vi "Sort Alarms.vi"(11 "alarms":T2(array[cluster])=[{"alarm URL"="\\\\Nate-VM-LV2018\\Pfizer_FAST_20190308T120351\\TT1.Alarms.TT1:Hi", "set time"=timestamp(3634909448.9887314 s since 1904-01-01), "set user"="(Nobody)", "ack time"=timestamp(-9223372036854775808 s since 1904-01-01), "ack user"="", "clear time"=timestamp(3634909450.4573107 s since 1904-01-01), "clear user"="(Nobody)", "setpoint"=70.0, "value"=70.46992251022208, "priority"=1, "alarm area"="", "alarm description"="", "ack comment"="", "event?"=FALSE, "Refnum"=216172782113784118}, {"alarm URL"="\\\\Nate-VM-LV2018\\Pfizer_FAST_20190308T120351\\TT1.Alarms.TT1:Hi", "set time"=timestamp(3634909451.127358 s since 1904-01-01), "set user"="(Nobody)", "ack time"=timestamp(-9223372036854775808 s since 1904-01-01), "ack user"="", "clear time"=timestamp(3634909453.4071665 s since 1904-01-01), "clear user"="(Nobody)", "setpoint"=70.0, "value"=71.57929385818943, "priority"=1, "alarm area"="", "alarm description"="", "ack comment"="", "event?"=FALSE, "Refnum"=216172782113784119}, {"alarm URL"="\\\\Nate-VM-LV2018\\Pfizer_FAST_20190308T120351\\TT1.Alarms.TT1:Hi", "set time"=timestamp(3634909453.907706 s since 1904-01-01), "set user"="(Nobody)", "ack time"=timestamp(-9223372036854775808 s since 1904-01-01), "ack user"="", "clear time"=timestamp(3634909456.7766027 s since 1904-01-01), "clear user"="(Nobody)", "setpoint"=70.0, "value"=71.76684506124857, "priority"=1, "alarm area"="", "alarm description"="", "ack comment"="", "event?"=FALSE, "Refnum"=216172782113784120}, {"alarm URL"="\\\\Nate-VM-LV2018\\Pfizer_FAST_20190308T120351\\TT1.Alarms.TT1:HiHi", "set time"=timestamp(3634909455.1962986 s since 1904-01-01), "set user"="(Nobody)", "ack time"=timestamp(-9223372036854775808 s since 1904-01-01), "ack user"="", "clear time"=timestamp(3634909456.1466627 s since 1904-01-01), "clear user"="(Nobody)", "setpoint"=80.0, "value"=80.61428399459591, "priority"=100, "alarm area"="", "alarm description"="", "ack comment"="", "event?"=FALSE, "Refnum"=216172782113784121}, {"alarm URL"="\\\\Nate-VM-LV2018\\Pfizer_FAST_20190308T120351\\TT1.Alarms.TT1:Hi", "set time"=timestamp(3634909457.266568 s since 1904-01-01), "set user"="(Nobody)", "ack time"=timestamp(-9223372036854775808 s since 1904-01-01), "ack user"="", "clear time"=timestamp(3634909458.256423 s since 1904-01-01), "clear user"="(Nobody)", "setpoint"=70.0, "value"=74.55000777818069, "priority"=1, "alarm area"="", "alarm description"="", "ack comment"="", "event?"=FALSE, "Refnum"=216172782113784122}, {"alarm URL"="\\\\Nate-VM-LV2018\\Pfizer_FAST_20190308T120351\\TT1.Alarms.TT1:HiHi", "set time"=timestamp(3634909457.306495 s since 1904-01-01), "set user"="(Nobody)", "ack time"=timestamp(-9223372036854775808 s since 1904-01-01), "ack user"="", "clear time"=timestamp(3634909457.716528 s since 1904-01-01), "clear user"="(Nobody)", "setpoint"=80.0, "value"=81.63729425968472, "priority"=100, "alarm area"="", "alarm description"="", "ack comment"="", "event?"=FALSE, "Refnum"=216172782113784123}, {"alarm URL"="\\\\Nate-VM-LV2018\\Pfizer_FAST_20190308T120351\\TT1.Alarms.TT1:HiHi", "set time"=timestamp(3634909457.9566164 s since 1904-01-01), "set user"="(Nobody)", "ack time"=timestamp(-9223372036854775808 s since 1904-01-01), "ack user"="", "clear time"=timestamp(3634909458.186914 s since 1904-01-01), "clear user"="(Nobody)", "setpoint"=80.0, "value"=80.37585970760009, "priority"=100, "alarm area"="", "alarm description"="", "ack comment"="", "event?"=FALSE, "Refnum"=216172782113784124}, {"alarm URL"="\\\\Nate-VM-LV2018\\Pfizer_FAST_20190308T120351\\TT1.Alarms.TT1:Hi", "set time"=timestamp(3634909458.776946 s since 1904-01-01), "set user"="(Nobody)", "ack time"=timestamp(-9223372036854775808 s since 1904-01-01), "ack user"="", "clear time"=timestamp(-9223372036854775808 s since 1904-01-01), "clear user"="", "setpoint"=70.0, "value"=71.54470210070821, "priority"=1, "alarm area"="", "alarm description"="", "ack comment"="", "event?"=FALSE, "Refnum"=216172782113784125}, {"alarm URL"="\\\\Nate-VM-LV2018\\Pfizer_FAST_20190308T120351\\TT1.Alarms.TT1:HiHi", "set time"=timestamp(3634909459.176953 s since 1904-01-01), "set user"="(Nobody)", "ack time"=timestamp(-9223372036854775808 s since 1904-01-01), "ack user"="", "clear time"=timestamp(3634909459.3466263 s since 1904-01-01), "clear user"="(Nobody)", "setpoint"=80.0, "value"=81.23368917949773, "priority"=100, "alarm area"="", "alarm description"="", "ack comment"="", "event?"=FALSE, "Refnum"=216172782113784126}, {"alarm URL"="\\\\Nate-VM-LV2018\\Pfizer_FAST_20190308T120351\\TT2.Alarms.TT2:Lo", "set time"=timestamp(3634909460.636917 s since 1904-01-01), "set user"="(Nobody)", "ack time"=timestamp(-9223372036854775808 s since 1904-01-01), "ack user"="", "clear time"=timestamp(3634909465.4269753 s since 1904-01-01), "clear user"="(Nobody)", "setpoint"=50.0, "value"=47.30826157706679, "priority"=1, "alarm area"="", "alarm description"="", "ack comment"="", "event?"=FALSE, "Refnum"=216172782113784127}, {"alarm URL"="\\\\Nate-VM-LV2018\\Pfizer_FAST_20190308T120351\\TT2.Alarms.TT2:LoLo", "set time"=timestamp(3634909461.5767922 s since 1904-01-01), "set user"="(Nobody)", "ack time"=timestamp(-9223372036854775808 s since 1904-01-01), "ack user"="", "clear time"=timestamp(3634909462.0770683 s since 1904-01-01), "clear user"="(Nobody)", "setpoint"=10.0, "value"=8.506791891117093, "priority"=100, "alarm area"="", "alarm description"="", "ack comment"="", "event?"=FALSE, "Refnum"=216172782113784128}, {"alarm URL"="\\\\Nate-VM-LV2018\\Pfizer_FAST_20190308T120351\\TT2.Alarms.TT2:LoLo", "set time"=timestamp(3634909462.2569776 s since 1904-01-01), "set user"="(Nobody)", "ack time"=timestamp(-9223372036854775808 s since 1904-01-01), "ack user"="", "clear time"=timestamp(3634909462.497084 s since 1904-01-01), "clear user"="(Nobody)", "setpoint"=10.0, "value"=4.924754519008068, "priority"=100, "alarm area"="", "alarm description"="", "ack comment"="", "event?"=FALSE, "Refnum"=216172782113784129}, {"alarm URL"="\\\\Nate-VM-LV2018\\Pfizer_FAST_20190308T120351\\TT2.Alarms.TT2:LoLo", "set time"=timestamp(3634909464.4868274 s since 1904-01-01), "set user"="(Nobody)", "ack time"=timestamp(-9223372036854775808 s since 1904-01-01), "ack user"="", "clear time"=timestamp(3634909464.6469216 s since 1904-01-01), "clear user"="(Nobody)", "setpoint"=10.0, "value"=8.582095188618679, "priority"=100, "alarm area"="", "alarm description"="", "ack comment"="", "event?"=FALSE, "Refnum"=216172782113784130}, {"alarm URL"="\\\\Nate-VM-LV2018\\Pfizer_FAST_20190308T120351\\TT2.Alarms.TT2:LoLo", "set time"=timestamp(3634909464.886837 s since 1904-01-01), "set user"="(Nobody)", "ack time"=timestamp(-9223372036854775808 s since 1904-01-01), "ack user"="", "clear time"=timestamp(3634909465.0468464 s since 1904-01-01), "clear user"="(Nobody)", "setpoint"=10.0, "value"=5.034174395850155, "priority"=100, "alarm area"="", "alarm description"="", "ack comment"="", "event?"=FALSE, "Refnum"=216172782113784131}] {"value" format="%.2f"; "setpoint" format="%.2f"; "clear time" format="%<%X\n%x>T"; "ack time" format="%<%X\n%x>T"; "set time" format="%<%X\n%x>T"}) -> (3 "alarms out":T2(array[cluster])=[{"alarm URL"="\\\\Nate-VM-LV2018\\Pfizer_FAST_20190308T120351\\TT1.Alarms.TT1:Hi", "set time"=timestamp(3634909458.776946 s since 1904-01-01), "set user"="(Nobody)", "ack time"=timestamp(-9223372036854775808 s since 1904-01-01), "ack user"="", "clear time"=timestamp(-9223372036854775808 s since 1904-01-01), "clear user"="", "setpoint"=70.0, "value"=71.54470210070821, "priority"=1, "alarm area"="", "alarm description"="", "ack comment"="", "event?"=FALSE, "Refnum"=216172782113784125}, {"alarm URL"="\\\\Nate-VM-LV2018\\Pfizer_FAST_20190308T120351\\TT2.Alarms.TT2:LoLo", "set time"=timestamp(3634909464.886837 s since 1904-01-01), "set user"="(Nobody)", "ack time"=timestamp(-9223372036854775808 s since 1904-01-01), "ack user"="", "clear time"=timestamp(3634909465.0468464 s since 1904-01-01), "clear user"="(Nobody)", "setpoint"=10.0, "value"=5.034174395850155, "priority"=100, "alarm area"="", "alarm description"="", "ack comment"="", "event?"=FALSE, "Refnum"=216172782113784131}, {"alarm URL"="\\\\Nate-VM-LV2018\\Pfizer_FAST_20190308T120351\\TT2.Alarms.TT2:LoLo", "set time"=timestamp(3634909464.4868274 s since 1904-01-01), "set user"="(Nobody)", "ack time"=timestamp(-9223372036854775808 s since 1904-01-01), "ack user"="", "clear time"=timestamp(3634909464.6469216 s since 1904-01-01), "clear user"="(Nobody)", "setpoint"=10.0, "value"=8.582095188618679, "priority"=100, "alarm area"="", "alarm description"="", "ack comment"="", "event?"=FALSE, "Refnum"=216172782113784130}, {"alarm URL"="\\\\Nate-VM-LV2018\\Pfizer_FAST_20190308T120351\\TT2.Alarms.TT2:LoLo", "set time"=timestamp(3634909462.2569776 s since 1904-01-01), "set user"="(Nobody)", "ack time"=timestamp(-9223372036854775808 s since 1904-01-01), "ack user"="", "clear time"=timestamp(3634909462.497084 s since 1904-01-01), "clear user"="(Nobody)", "setpoint"=10.0, "value"=4.924754519008068, "priority"=100, "alarm area"="", "alarm description"="", "ack comment"="", "event?"=FALSE, "Refnum"=216172782113784129}, {"alarm URL"="\\\\Nate-VM-LV2018\\Pfizer_FAST_20190308T120351\\TT2.Alarms.TT2:LoLo", "set time"=timestamp(3634909461.5767922 s since 1904-01-01), "set user"="(Nobody)", "ack time"=timestamp(-9223372036854775808 s since 1904-01-01), "ack user"="", "clear time"=timestamp(3634909462.0770683 s since 1904-01-01), "clear user"="(Nobody)", "setpoint"=10.0, "value"=8.506791891117093, "priority"=100, "alarm area"="", "alarm description"="", "ack comment"="", "event?"=FALSE, "Refnum"=216172782113784128}, {"alarm URL"="\\\\Nate-VM-LV2018\\Pfizer_FAST_20190308T120351\\TT1.Alarms.TT1:HiHi", "set time"=timestamp(3634909459.176953 s since 1904-01-01), "set user"="(Nobody)", "ack time"=timestamp(-9223372036854775808 s since 1904-01-01), "ack user"="", "clear time"=timestamp(3634909459.3466263 s since 1904-01-01), "clear user"="(Nobody)", "setpoint"=80.0, "value"=81.23368917949773, "priority"=100, "alarm area"="", "alarm description"="", "ack comment"="", "event?"=FALSE, "Refnum"=216172782113784126}, {"alarm URL"="\\\\Nate-VM-LV2018\\Pfizer_FAST_20190308T120351\\TT1.Alarms.TT1:HiHi", "set time"=timestamp(3634909457.9566164 s since 1904-01-01), "set user"="(Nobody)", "ack time"=timestamp(-9223372036854775808 s since 1904-01-01), "ack user"="", "clear time"=timestamp(3634909458.186914 s since 1904-01-01), "clear user"="(Nobody)", "setpoint"=80.0, "value"=80.37585970760009, "priority"=100, "alarm area"="", "alarm description"="", "ack comment"="", "event?"=FALSE, "Refnum"=216172782113784124}, {"alarm URL"="\\\\Nate-VM-LV2018\\Pfizer_FAST_20190308T120351\\TT1.Alarms.TT1:HiHi", "set time"=timestamp(3634909457.306495 s since 1904-01-01), "set user"="(Nobody)", "ack time"=timestamp(-9223372036854775808 s since 1904-01-01), "ack user"="", "clear time"=timestamp(3634909457.716528 s since 1904-01-01), "clear user"="(Nobody)", "setpoint"=80.0, "value"=81.63729425968472, "priority"=100, "alarm area"="", "alarm description"="", "ack comment"="", "event?"=FALSE, "Refnum"=216172782113784123}, {"alarm URL"="\\\\Nate-VM-LV2018\\Pfizer_FAST_20190308T120351\\TT1.Alarms.TT1:HiHi", "set time"=timestamp(3634909455.1962986 s since 1904-01-01), "set user"="(Nobody)", "ack time"=timestamp(-9223372036854775808 s since 1904-01-01), "ack user"="", "clear time"=timestamp(3634909456.1466627 s since 1904-01-01), "clear user"="(Nobody)", "setpoint"=80.0, "value"=80.61428399459591, "priority"=100, "alarm area"="", "alarm description"="", "ack comment"="", "event?"=FALSE, "Refnum"=216172782113784121}, {"alarm URL"="\\\\Nate-VM-LV2018\\Pfizer_FAST_20190308T120351\\TT2.Alarms.TT2:Lo", "set time"=timestamp(3634909460.636917 s since 1904-01-01), "set user"="(Nobody)", "ack time"=timestamp(-9223372036854775808 s since 1904-01-01), "ack user"="", "clear time"=timestamp(3634909465.4269753 s since 1904-01-01), "clear user"="(Nobody)", "setpoint"=50.0, "value"=47.30826157706679, "priority"=1, "alarm area"="", "alarm description"="", "ack comment"="", "event?"=FALSE, "Refnum"=216172782113784127}, {"alarm URL"="\\\\Nate-VM-LV2018\\Pfizer_FAST_20190308T120351\\TT1.Alarms.TT1:Hi", "set time"=timestamp(3634909457.266568 s since 1904-01-01), "set user"="(Nobody)", "ack time"=timestamp(-9223372036854775808 s since 1904-01-01), "ack user"="", "clear time"=timestamp(3634909458.256423 s since 1904-01-01), "clear user"="(Nobody)", "setpoint"=70.0, "value"=74.55000777818069, "priority"=1, "alarm area"="", "alarm description"="", "ack comment"="", "event?"=FALSE, "Refnum"=216172782113784122}, {"alarm URL"="\\\\Nate-VM-LV2018\\Pfizer_FAST_20190308T120351\\TT1.Alarms.TT1:Hi", "set time"=timestamp(3634909453.907706 s since 1904-01-01), "set user"="(Nobody)", "ack time"=timestamp(-9223372036854775808 s since 1904-01-01), "ack user"="", "clear time"=timestamp(3634909456.7766027 s since 1904-01-01), "clear user"="(Nobody)", "setpoint"=70.0, "value"=71.76684506124857, "priority"=1, "alarm area"="", "alarm description"="", "ack comment"="", "event?"=FALSE, "Refnum"=216172782113784120}, {"alarm URL"="\\\\Nate-VM-LV2018\\Pfizer_FAST_20190308T120351\\TT1.Alarms.TT1:Hi", "set time"=timestamp(3634909451.127358 s since 1904-01-01), "set user"="(Nobody)", "ack time"=timestamp(-9223372036854775808 s since 1904-01-01), "ack user"="", "clear time"=timestamp(3634909453.4071665 s since 1904-01-01), "clear user"="(Nobody)", "setpoint"=70.0, "value"=71.57929385818943, "priority"=1, "alarm area"="", "alarm description"="", "ack comment"="", "event?"=FALSE, "Refnum"=216172782113784119}, {"alarm URL"="\\\\Nate-VM-LV2018\\Pfizer_FAST_20190308T120351\\TT1.Alarms.TT1:Hi", "set time"=timestamp(3634909448.9887314 s since 1904-01-01), "set user"="(Nobody)", "ack time"=timestamp(-9223372036854775808 s since 1904-01-01), "ack user"="", "clear time"=timestamp(3634909450.4573107 s since 1904-01-01), "clear user"="(Nobody)", "setpoint"=70.0, "value"=70.46992251022208, "priority"=1, "alarm area"="", "alarm description"="", "ack comment"="", "event?"=FALSE, "Refnum"=216172782113784118}] {"value" format="%.2f"; "setpoint" format="%.2f"; "clear time" format="%<%X\n%x>T"; "ack time" format="%<%X\n%x>T"; "set time" format="%<%X\n%x>T"})   [LabVIEW 2018, in "Dynamic Shared Variables.lvlib"]
doc: "Sort alarms per Delta V alarm ranking."
uses:
  Dynamic Shared Variables.lvlib
panel:
  out "Array":T1(array[cluster])=[{113635.90945877694604, "Alarm"={"alarm URL"="\\\\Nate-VM-LV2018\\Pfizer_FAST_20190308T120351\\TT1.Alarms.TT1:Hi", "set time"=timestamp(3634909458.776946 s since 1904-01-01), "set user"="(Nobody)", "ack time"=timestamp(-9223372036854775808 s since 1904-01-01), "ack user"="", "clear time"=timestamp(-9223372036854775808 s since 1904-01-01), "clear user"="", "setpoint"=70.0, "value"=71.54470210070821, "priority"=1, "alarm area"="", "alarm description"="", "ack comment"="", "event?"=FALSE, "Refnum"=216172782113784125}}, {103734.909464886837036, "Alarm"={"alarm URL"="\\\\Nate-VM-LV2018\\Pfizer_FAST_20190308T120351\\TT2.Alarms.TT2:LoLo", "set time"=timestamp(3634909464.886837 s since 1904-01-01), "set user"="(Nobody)", "ack time"=timestamp(-9223372036854775808 s since 1904-01-01), "ack user"="", "clear time"=timestamp(3634909465.0468464 s since 1904-01-01), "clear user"="(Nobody)", "setpoint"=10.0, "value"=5.034174395850155, "priority"=100, "alarm area"="", "alarm description"="", "ack comment"="", "event?"=FALSE, "Refnum"=216172782113784131}}, {103734.909464486827133, "Alarm"={"alarm URL"="\\\\Nate-VM-LV2018\\Pfizer_FAST_20190308T120351\\TT2.Alarms.TT2:LoLo", "set time"=timestamp(3634909464.4868274 s since 1904-01-01), "set user"="(Nobody)", "ack time"=timestamp(-9223372036854775808 s since 1904-01-01), "ack user"="", "clear time"=timestamp(3634909464.6469216 s since 1904-01-01), "clear user"="(Nobody)", "setpoint"=10.0, "value"=8.582095188618679, "priority"=100, "alarm area"="", "alarm description"="", "ack comment"="", "event?"=FALSE, "Refnum"=216172782113784130}}, {103734.909462256977434, "Alarm"={"alarm URL"="\\\\Nate-VM-LV2018\\Pfizer_FAST_20190308T120351\\TT2.Alarms.TT2:LoLo", "set time"=timestamp(3634909462.2569776 s since 1904-01-01), "set user"="(Nobody)", "ack time"=timestamp(-9223372036854775808 s since 1904-01-01), "ack user"="", "clear time"=timestamp(3634909462.497084 s since 1904-01-01), "clear user"="(Nobody)", "setpoint"=10.0, "value"=4.924754519008068, "priority"=100, "alarm area"="", "alarm description"="", "ack comment"="", "event?"=FALSE, "Refnum"=216172782113784129}}, {103734.909461576791934, "Alarm"={"alarm URL"="\\\\Nate-VM-LV2018\\Pfizer_FAST_20190308T120351\\TT2.Alarms.TT2:LoLo", "set time"=timestamp(3634909461.5767922 s since 1904-01-01), "set user"="(Nobody)", "ack time"=timestamp(-9223372036854775808 s since 1904-01-01), "ack user"="", "clear time"=timestamp(3634909462.0770683 s since 1904-01-01), "clear user"="(Nobody)", "setpoint"=10.0, "value"=8.506791891117093, "priority"=100, "alarm area"="", "alarm description"="", "ack comment"="", "event?"=FALSE, "Refnum"=216172782113784128}}, {103734.909459176952836, "Alarm"={"alarm URL"="\\\\Nate-VM-LV2018\\Pfizer_FAST_20190308T120351\\TT1.Alarms.TT1:HiHi", "set time"=timestamp(3634909459.176953 s since 1904-01-01), "set user"="(Nobody)", "ack time"=timestamp(-9223372036854775808 s since 1904-01-01), "ack user"="", "clear time"=timestamp(3634909459.3466263 s since 1904-01-01), "clear user"="(Nobody)", "setpoint"=80.0, "value"=81.23368917949773, "priority"=100, "alarm area"="", "alarm description"="", "ack comment"="", "event?"=FALSE, "Refnum"=216172782113784126}}, {103734.909457956616237, "Alarm"={"alarm URL"="\\\\Nate-VM-LV2018\\Pfizer_FAST_20190308T120351\\TT1.Alarms.TT1:HiHi", "set time"=timestamp(3634909457.9566164 s since 1904-01-01), "set user"="(Nobody)", "ack time"=timestamp(-9223372036854775808 s since 1904-01-01), "ack user"="", "clear time"=timestamp(3634909458.186914 s since 1904-01-01), "clear user"="(Nobody)", "setpoint"=80.0, "value"=80.37585970760009, "priority"=100, "alarm area"="", "alarm description"="", "ack comment"="", "event?"=FALSE, "Refnum"=216172782113784124}}, {103734.909457306494836, "Alarm"={"alarm URL"="\\\\Nate-VM-LV2018\\Pfizer_FAST_20190308T120351\\TT1.Alarms.TT1:HiHi", "set time"=timestamp(3634909457.306495 s since 1904-01-01), "set user"="(Nobody)", "ack time"=timestamp(-9223372036854775808 s since 1904-01-01), "ack user"="", "clear time"=timestamp(3634909457.716528 s since 1904-01-01), "clear user"="(Nobody)", "setpoint"=80.0, "value"=81.63729425968472, "priority"=100, "alarm area"="", "alarm description"="", "ack comment"="", "event?"=FALSE, "Refnum"=216172782113784123}}, {103734.90945519629844, "Alarm"={"alarm URL"="\\\\Nate-VM-LV2018\\Pfizer_FAST_20190308T120351\\TT1.Alarms.TT1:HiHi", "set time"=timestamp(3634909455.1962986 s since 1904-01-01), "set user"="(Nobody)", "ack time"=timestamp(-9223372036854775808 s since 1904-01-01), "ack user"="", "clear time"=timestamp(3634909456.1466627 s since 1904-01-01), "clear user"="(Nobody)", "setpoint"=80.0, "value"=80.61428399459591, "priority"=100, "alarm area"="", "alarm description"="", "ack comment"="", "event?"=FALSE, "Refnum"=216172782113784121}}, {103635.90946063691693, "Alarm"={"alarm URL"="\\\\Nate-VM-LV2018\\Pfizer_FAST_20190308T120351\\TT2.Alarms.TT2:Lo", "set time"=timestamp(3634909460.636917 s since 1904-01-01), "set user"="(Nobody)", "ack time"=timestamp(-9223372036854775808 s since 1904-01-01), "ack user"="", "clear time"=timestamp(3634909465.4269753 s since 1904-01-01), "clear user"="(Nobody)", "setpoint"=50.0, "value"=47.30826157706679, "priority"=1, "alarm area"="", "alarm description"="", "ack comment"="", "event?"=FALSE, "Refnum"=216172782113784127}}, {103635.909457266567834, "Alarm"={"alarm URL"="\\\\Nate-VM-LV2018\\Pfizer_FAST_20190308T120351\\TT1.Alarms.TT1:Hi", "set time"=timestamp(3634909457.266568 s since 1904-01-01), "set user"="(Nobody)", "ack time"=timestamp(-9223372036854775808 s since 1904-01-01), "ack user"="", "clear time"=timestamp(3634909458.256423 s since 1904-01-01), "clear user"="(Nobody)", "setpoint"=70.0, "value"=74.55000777818069, "priority"=1, "alarm area"="", "alarm description"="", "ack comment"="", "event?"=FALSE, "Refnum"=216172782113784122}}, {103635.90945390770563, "Alarm"={"alarm URL"="\\\\Nate-VM-LV2018\\Pfizer_FAST_20190308T120351\\TT1.Alarms.TT1:Hi", "set time"=timestamp(3634909453.907706 s since 1904-01-01), "set user"="(Nobody)", "ack time"=timestamp(-9223372036854775808 s since 1904-01-01), "ack user"="", "clear time"=timestamp(3634909456.7766027 s since 1904-01-01), "clear user"="(Nobody)", "setpoint"=70.0, "value"=71.76684506124857, "priority"=1, "alarm area"="", "alarm description"="", "ack comment"="", "event?"=FALSE, "Refnum"=216172782113784120}}, {103635.909451127357734, "Alarm"={"alarm URL"="\\\\Nate-VM-LV2018\\Pfizer_FAST_20190308T120351\\TT1.Alarms.TT1:Hi", "set time"=timestamp(3634909451.127358 s since 1904-01-01), "set user"="(Nobody)", "ack time"=timestamp(-9223372036854775808 s since 1904-01-01), "ack user"="", "clear time"=timestamp(3634909453.4071665 s since 1904-01-01), "clear user"="(Nobody)", "setpoint"=70.0, "value"=71.57929385818943, "priority"=1, "alarm area"="", "alarm description"="", "ack comment"="", "event?"=FALSE, "Refnum"=216172782113784119}}, {103635.909448988731135, "Alarm"={"alarm URL"="\\\\Nate-VM-LV2018\\Pfizer_FAST_20190308T120351\\TT1.Alarms.TT1:Hi", "set time"=timestamp(3634909448.9887314 s since 1904-01-01), "set user"="(Nobody)", "ack time"=timestamp(-9223372036854775808 s since 1904-01-01), "ack user"="", "clear time"=timestamp(3634909450.4573107 s since 1904-01-01), "clear user"="(Nobody)", "setpoint"=70.0, "value"=70.46992251022208, "priority"=1, "alarm area"="", "alarm description"="", "ack comment"="", "event?"=FALSE, "Refnum"=216172782113784118}}]
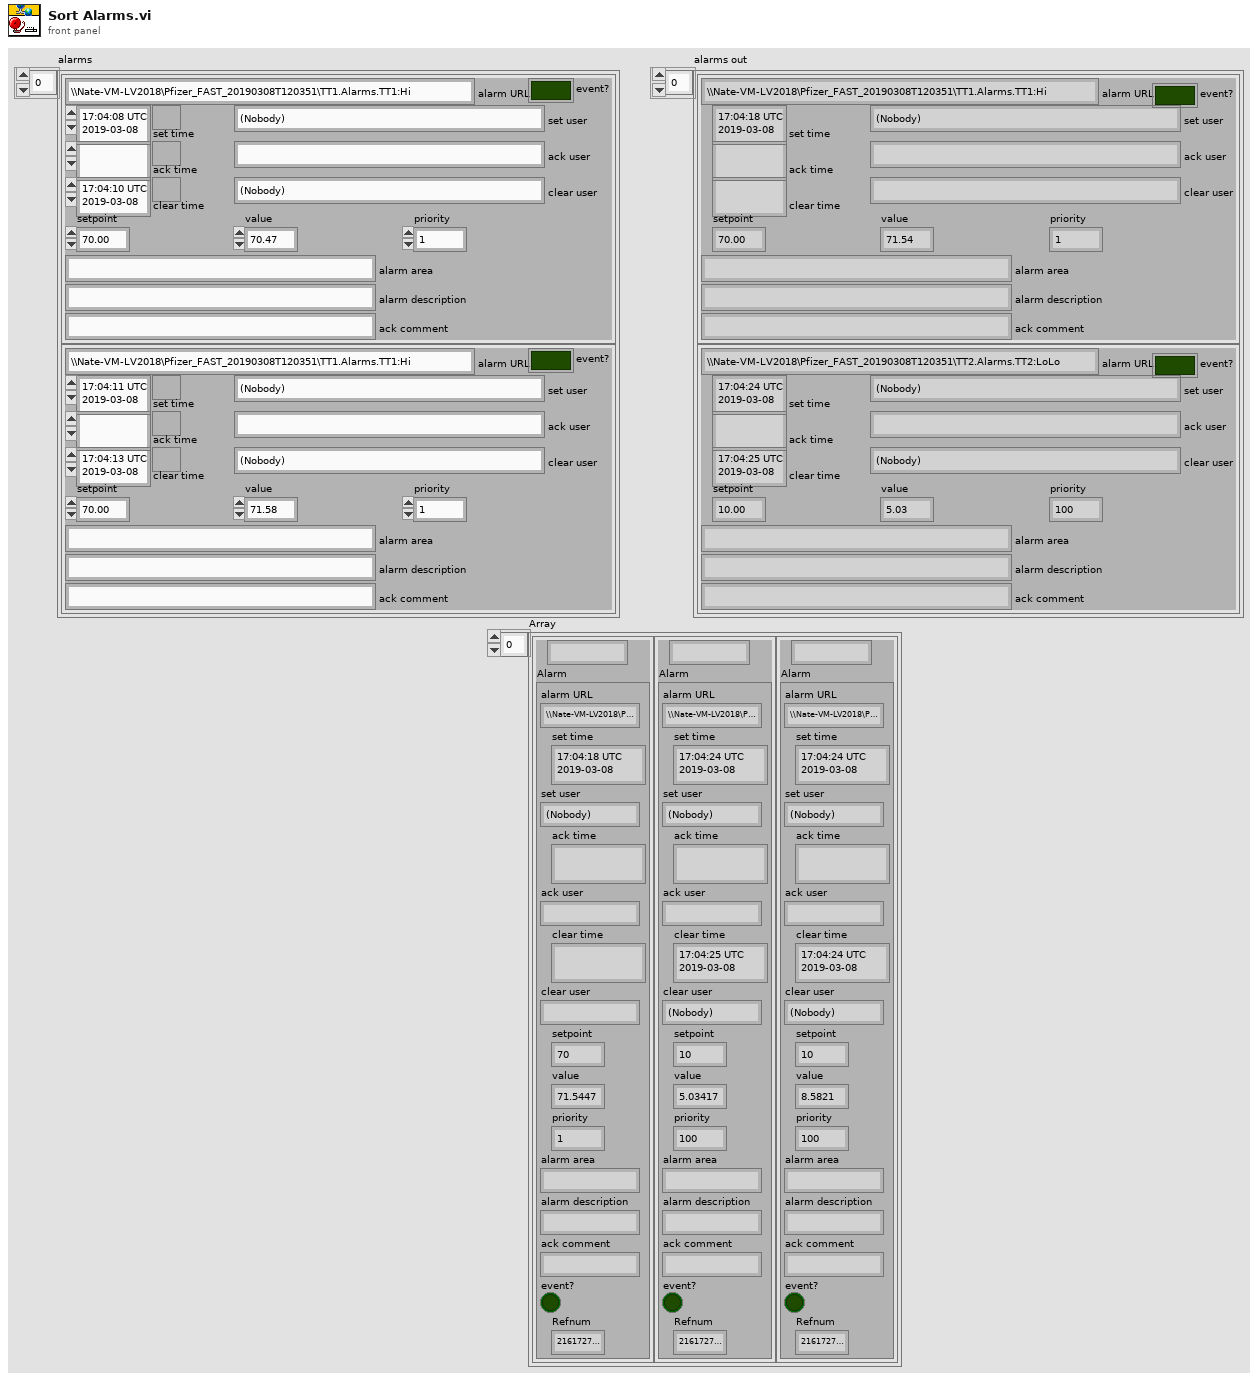
[diagram p1: front panel]
types:
  T1 = cluster{ext, "Alarm":cluster{"alarm URL":string, "set time":timestamp, "set user":string, "ack time":timestamp, "ack user":string, "clear time":timestamp, "clear user":string, "setpoint":dbl, "value":dbl, "priority":u32, "alarm area":string, "alarm description":string, "ack comment":string, "event?":bool, "Refnum":u64}}[]
  T2 = cluster{"alarm URL":string, "set time":timestamp, "set user":string, "ack time":timestamp, "ack user":string, "clear time":timestamp, "clear user":string, "setpoint":dbl, "value":dbl, "priority":u32, "alarm area":string, "alarm description":string, "ack comment":string, "event?":bool, "Refnum":u64}[]
  T3 = cluster{ext, "Alarm":cluster{"alarm URL":string, "set time":timestamp, "set user":string, "ack time":timestamp, "ack user":string, "clear time":timestamp, "clear user":string, "setpoint":dbl, "value":dbl, "priority":u32, "alarm area":string, "alarm description":string, "ack comment":string, "event?":bool, "Refnum":u64}}
  T4 = cluster{"alarm URL":string, "set time":timestamp, "set user":string, "ack time":timestamp, "ack user":string, "clear time":timestamp, "clear user":string, "setpoint":dbl, "value":dbl, "priority":u32, "alarm area":string, "alarm description":string, "ack comment":string, "event?":bool, "Refnum":u64}
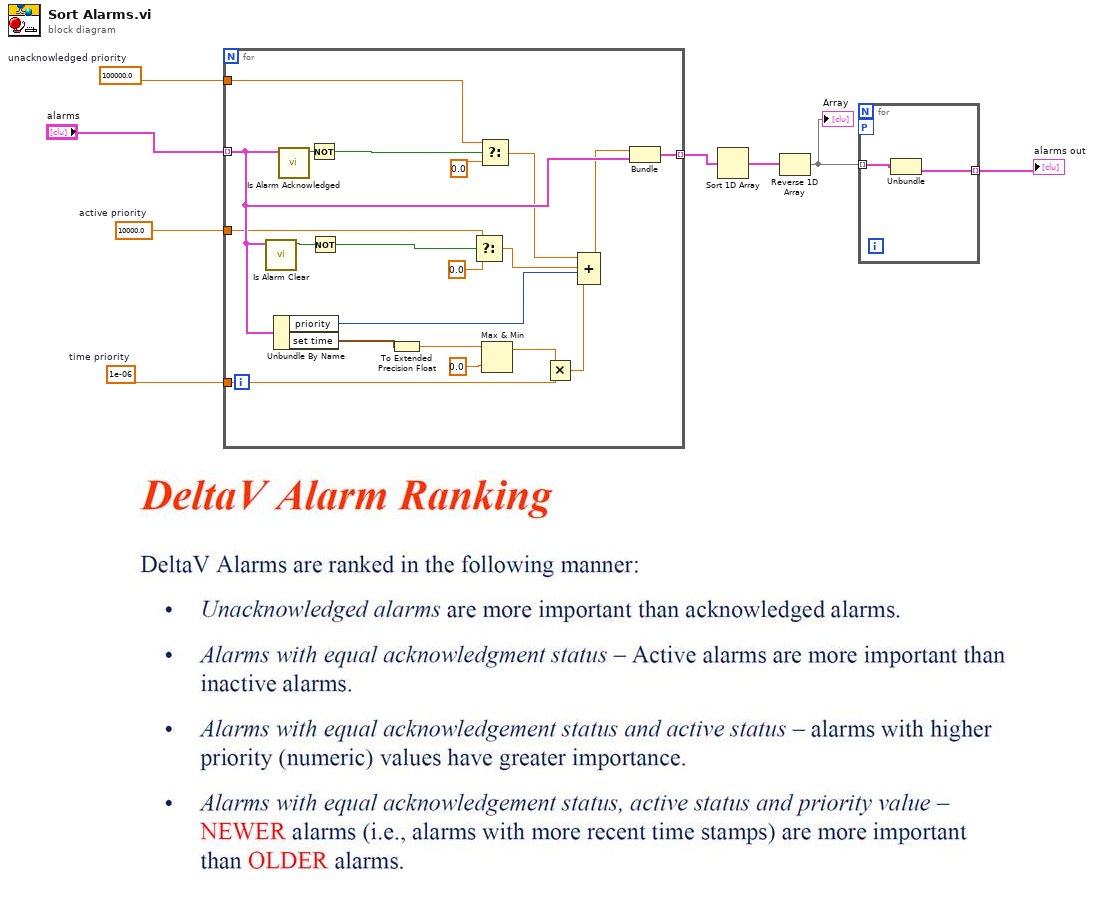
[diagram p0: block diagram]
diagram:
  w5 = 1e-06  # time priority
  w6 = 10000.0  # active priority
  w7 = 100000.0  # unacknowledged priority
  n1 = for {
    tunnel: "alarms" -> [w27] mode=indexing
    tunnel: w7 -> [w22]
    tunnel: w6 -> [w26]
    tunnel: w5 -> [w14]
    tunnel: [w10] -> w4 mode=indexing
    n2 = call "Is Alarm Clear.vi"("Alarm"=w27) -> ("Cleared?"=w25:bool)  [unwired: 10 in]
    n3 = Unbundle By Name(w27) -> ("priority"=w18:u32, "set time"=w16:timestamp)
    n4 = call "Is Alarm Acknowledged.vi"("Alarm"=w27) -> ("Acknowledged?"=w28:bool)  [unwired: 8 in, 2 out]
    n5 = Not(x=w28) -> (.not. x?=w24:bool)
    n6 = Not(x=w25) -> (.not. x?=w9:bool)
    n7 = To Extended Precision Float(1:w16) -> (0:w15:ext)
    n8 = Select(t=w26, s=w9, f=0.0 ("t")) -> (s? t:f=w19:dbl)
    n9 = Select(t=w22, s=w24, f=0.0 ("t")) -> (s? t:f=w20:dbl)
    n10 = Max & Min(x=w15, y=0.0 ("t")) -> (max(x,y)=w13:ext)  [unwired: 1 out]
    n11 = Multiply(x=w13, y=w14) -> (x*y=w12:ext)
    n12 = Compound Arithmetic op=ADD(w20, w19, w18, w12) -> (w11:ext)
    n13 = Bundle(w11, "Alarm"=w27) -> (w10:T3)  [unwired: 1 in]
  }
  n14 = Sort 1D Array(array=w4) -> (sorted array=w3:T1)
  n15 = Reverse 1D Array(array=w3) -> (reversed array=w1:T1)
  "Array" <- w1
  n16 = for {
    tunnel: w1 -> [w30] mode=indexing
    tunnel: [w29] -> w2 mode=indexing
    workers-P: _ -> [_]
    n17 = Unbundle(w30) -> ("Alarm"=w29:T4)  [unwired: 1 out]
  }
  "alarms out" <- w2
